vi "Position.vi"() -> (2 "Positions":T1 {"z (mm)" format="%.1p"; "y (nm)" format="%.1p"; "x (nm)" format="%.1p"})   [LabVIEW 2017]
uses:
  Program Files/National Instruments/LabVIEW 2019/user.lib/HapticSTM/HapticSTM.lvlib
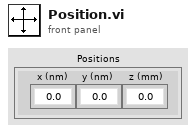
[diagram p1: front panel]
types:
  T1 = cluster{"x (nm)":dbl, "y (nm)":dbl, "z (mm)":dbl}
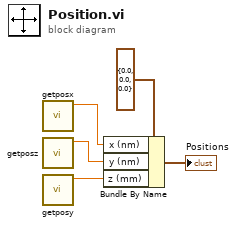
[diagram p0: block diagram]
diagram:
  n1 = call "getposx.vi"() -> ("function return"=w3:dbl)  [unwired: 11 in]
  n2 = call "getposz.vi"() -> ("function return"=w2:dbl)  [unwired: 11 in]
  n3 = call "getposy.vi"() -> ("function return"=w1:dbl)  [unwired: 11 in]
  n4 = Bundle By Name(cluster=T1 {"x (nm)"=0.0, "y (nm)"=0.0, "z (mm)"=0.0} ("Positions"), "x (nm)"=w3, "y (nm)"=w2, "z (mm)"=w1) -> (→"Positions":T1)
